vi "Vision Processing.vi"(4 "error in (no error)":errorcluster, 7 "Image Size":T6=enum."320x240") -> ()   [LabVIEW 2015]
doc: "This VI runs in parallel to other tasks. It gets images from the camera, processes them for color or shape and use that information to affect robot behavior."
uses:
  <vilib>/Rock Robotics/WPI/Camera/WPI_CameraImageSize.ctl
  examples/Vision Support Code/Camera Types.ctl
  <vilib>/Rock Robotics/WPI/Camera/WPI_CameraWhite Balance Values.ctl
  <vilib>/Rock Robotics/WPI/Camera/WPI_CameraExposure Values.ctl
  <vilib>/Rock Robotics/WPI/Camera/WPI_CameraFrameRate.ctl
  Robot Global Data.vi
  <vilib>/vision/NI_Vision_Development_Module.lvlib
  <vilib>/Rock Robotics/Network Tables/NT Read Numeric Array.vi
panel:
  in  "Right Boundary":dbl=0.07
  in  "Left Boundary":dbl=-0.07
  out "Centering Command":enum16{"NULL", "RIGHT", "LEFT", "CENTER"}(ring)
  out "Horizontal Centering":dbl
  out "fps":dbl
  in  "LED Color":T1={"Hue"={97.8946764540238, 78.89044183841362}, "Sat"={182.14285714285714, 255.0}, "Val"={106.25, 255.0}} {"Hue" scale=0.0..255.0 scale format="%#_3g"}
  out "Qualified Particles":i32
  in  "Score Threshold":dbl=75.0
  in  "Aspect Fudge Factor":dbl=1.0
  in  "Min Score Threshold":i32=75
  in  "Camera Type":T2=enum."1011"
  in  "Emphasize Limit Tests":bool=TRUE
  out "Masked":T3(plugin-control)
  in  "Display Mask":bool=TRUE
  out "Original Image":T3(plugin-control)
  in  "Display Original":bool=TRUE
  out "Sorted Particle Scores":T4(array[cluster]) {"Moment Factor" format="%#_3g"; "Aspect Ratio" format="%#_3g"; "Area to CH" format="%#_3g"; "X" format="%#_3g"; "Y" format="%#_3g"}
  out "Highest Avg Score":dbl
  out "Detected Targets":T5(array[cluster]) {"Normalized Rect"."Numeric 5" format="%#_2g"; "Normalized Rect"."Numeric 3" format="%#_2g"; "Normalized Rect"."Numeric 2" format="%#_2g"; "Normalized Rect"."Numeric" format="%#_2g"}
  out "ms to process":u32
  # "Density Profile"
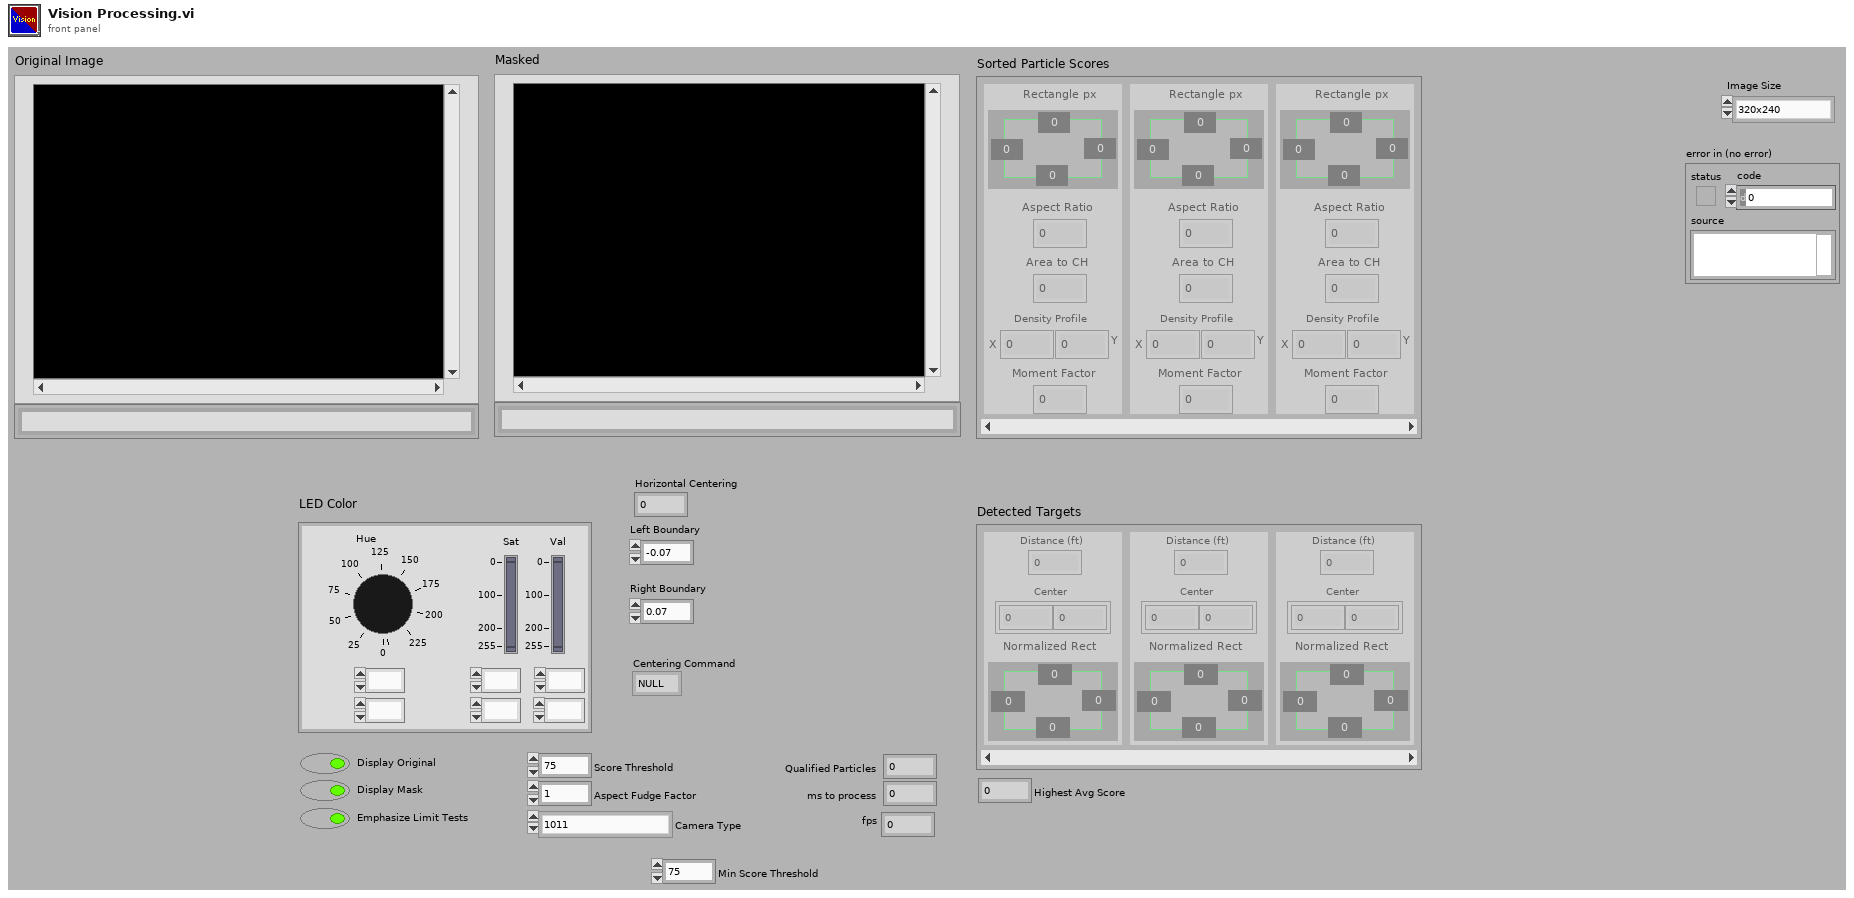
[diagram p1: front panel]
types:
  T1 = cluster{"Hue":cluster{dbl, dbl}, "Sat":cluster{dbl, dbl}, "Val":cluster{dbl, dbl}}
  T2 = typedef "Camera Types.ctl" = enum16{"206", "1011", "1013", "MS HD3000 square", "MS HD3000 640x480"}
  T3 = typedef "IMAQ Image.ctl" = refnum<image>
  T4 = cluster{"Rectangle px":cluster{"Numeric":dbl, "Numeric 2":dbl, "Numeric 3":dbl, "Numeric 5":dbl}, "Aspect Ratio":dbl, "Area to CH":dbl, "X":dbl, "Y":dbl, "Moment Factor":dbl}[]
  T5 = cluster{"Distance (ft)":dbl, "Center":cluster{dbl, dbl}, "Normalized Rect":cluster{"Numeric":dbl, "Numeric 2":dbl, "Numeric 3":dbl, "Numeric 5":dbl}}[]
  T6 = typedef "WPI_CameraImageSize.ctl" = enum16{"640x480", "320x240", "160x120", "Custom"}
  T7 = typedef "Particle Parameters" = i32
  T8 = typedef "WPI_CameraFrameRate.ctl" = u32
  T9 = typedef "WPI_CameraExposure Values.ctl" = enum16{"Auto", "Flicker-free 50 Hz", "Flicker-free 60 Hz", "Hold current", "Custom"}
  T10 = typedef "WPI_CameraWhite Balance Values.ctl" = enum16{"Auto", "Fixed indoor", "Fixed outdoor 1", "Fixed outdoor 2", "Fixed fluorescent 1", "Fixed fluorescent 2", "Hold current", "Custom"}
  T11 = typedef "Image Type" = u32
  T12 = typedef "WPI_CameraDevRef.ctl" = cluster{"Camera Address":string, "CameraStatus":errorcluster}
  T13 = cluster{"Numeric Array[0]":dbl, "Numeric Array[1]":dbl, "Numeric Array[2]":dbl, "Numeric Array[3]":dbl, "Numeric Array[4]":dbl, "Numeric Array[5]":dbl, "Numeric Array[6]":dbl, "Numeric Array[7]":dbl, "Numeric Array[8]":dbl}
  T14 = cluster{"Bounding box":cluster{"left":dbl, "top":dbl, "right":dbl, "bottom":dbl}, "Aspect Ratio":dbl, "Area to CH":dbl, "X Mask":dbl, "Y Mask":dbl, "Moment":dbl}[]
  T15 = cluster{"Rectangle":cluster{"Numeric":dbl, "Numeric 2":dbl, "Numeric 3":dbl, "Numeric 5":dbl}, "L":dbl, "Area to CH":dbl, "X":dbl, "Y":dbl, "Moment Factor":dbl}[]
  T16 = cluster{"Found Targets[0]":cluster{"Distance (ft)":dbl, "Center":cluster{dbl, dbl}, "Normalized Rect":cluster{"Numeric":dbl, "Numeric 2":dbl, "Numeric 3":dbl, "Numeric 5":dbl}}, "Found Targets[1]":cluster{"Distance (ft)":dbl, "Center":cluster{dbl, dbl}, "Normalized Rect":cluster{"Numeric":dbl, "Numeric 2":dbl, "Numeric 3":dbl, "Numeric 5":dbl}}, "Found Targets[2]":cluster{"Distance (ft)":dbl, "Center":cluster{dbl, dbl}, "Normalized Rect":cluster{"Numeric":dbl, "Numeric 2":dbl, "Numeric 3":dbl, "Numeric 5":dbl}}, "Found Targets[3]":cluster{"Distance (ft)":dbl, "Center":cluster{dbl, dbl}, "Normalized Rect":cluster{"Numeric":dbl, "Numeric 2":dbl, "Numeric 3":dbl, "Numeric 5":dbl}}, "Found Targets[4]":cluster{"Distance (ft)":dbl, "Center":cluster{dbl, dbl}, "Normalized Rect":cluster{"Numeric":dbl, "Numeric 2":dbl, "Numeric 3":dbl, "Numeric 5":dbl}}, "Found Targets[5]":cluster{"Distance (ft)":dbl, "Center":cluster{dbl, dbl}, "Normalized Rect":cluster{"Numeric":dbl, "Numeric 2":dbl, "Numeric 3":dbl, "Numeric 5":dbl}}, "Found Targets[6]":cluster{"Distance (ft)":dbl, "Center":cluster{dbl, dbl}, "Normalized Rect":cluster{"Numeric":dbl, "Numeric 2":dbl, "Numeric 3":dbl, "Numeric 5":dbl}}, "Found Targets[7]":cluster{"Distance (ft)":dbl, "Center":cluster{dbl, dbl}, "Normalized Rect":cluster{"Numeric":dbl, "Numeric 2":dbl, "Numeric 3":dbl, "Numeric 5":dbl}}, "Found Targets[8]":cluster{"Distance (ft)":dbl, "Center":cluster{dbl, dbl}, "Normalized Rect":cluster{"Numeric":dbl, "Numeric 2":dbl, "Numeric 3":dbl, "Numeric 5":dbl}}}
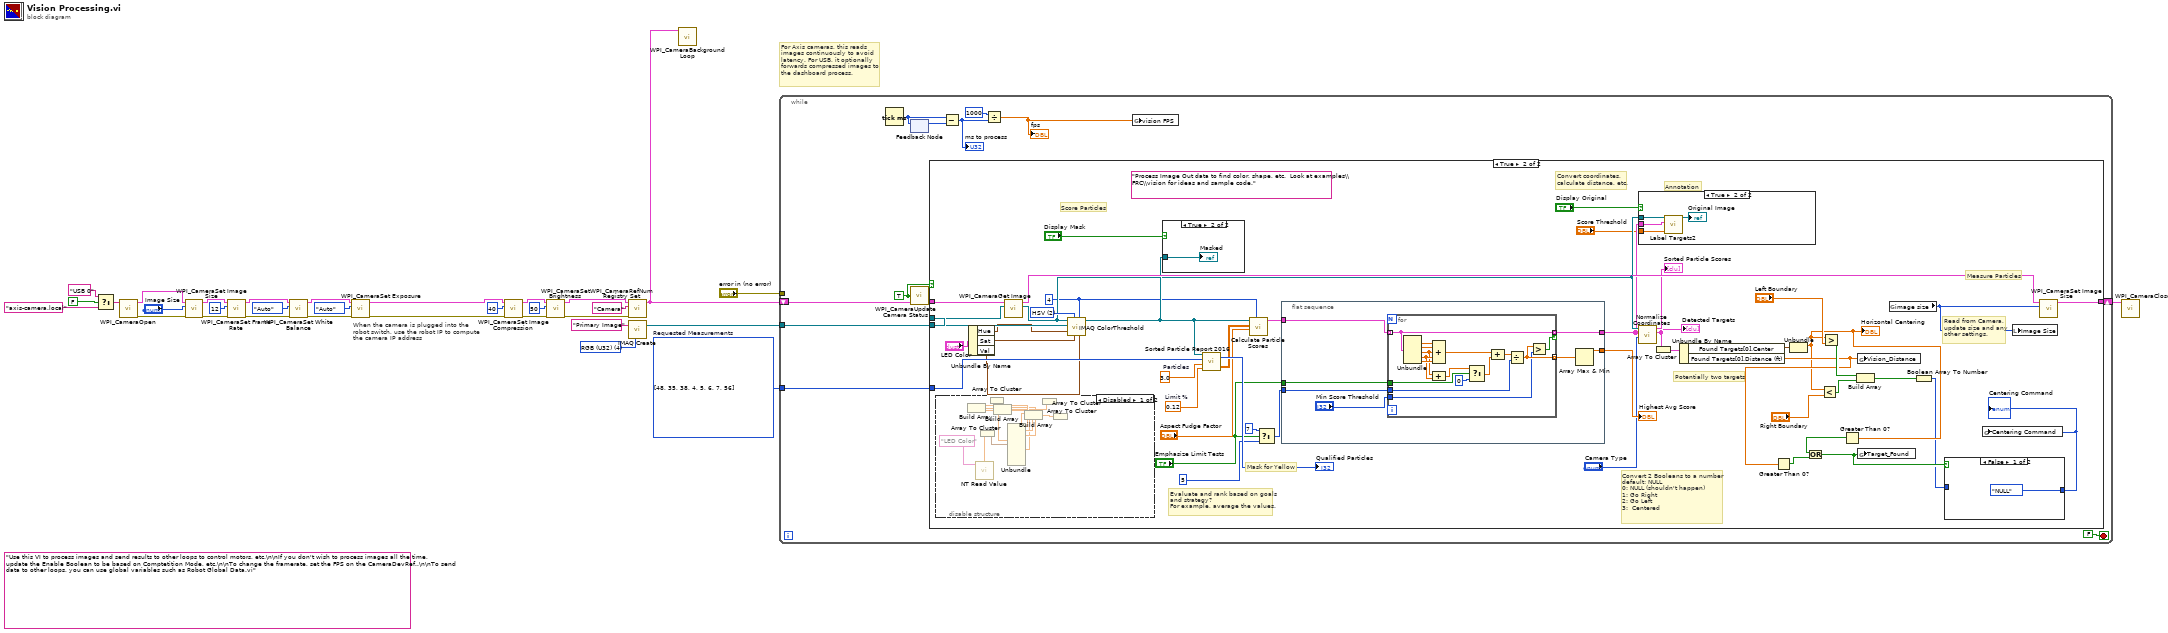
[diagram p0: block diagram]
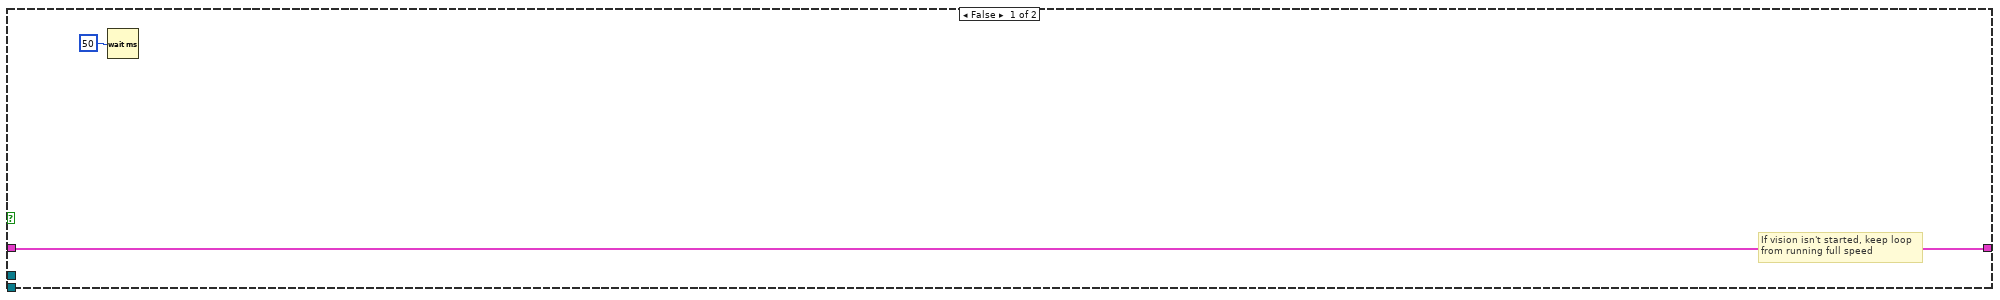
[diagram p2: hidden frame]
diagram:
  w1 = T7[] [48, 35, 38, 4, 5, 6, 7, 56] items=["Center of Mass X", "Center of Mass Y", "First Pixel X", "First Pixel Y", "Bounding Rect Left", "Bounding Rect Top", "Bounding Rect Right", "Bounding Rect Bottom", "Max Feret Diameter Start X", "Max Feret Diameter Start Y", "Max Feret Diameter End X", "Max Feret Diameter End Y", "Max Horiz. Segment Length Left", "Max Horiz. Segment Length Right", "Max Horiz. Segment Length Row", "-", "Bounding Rect Width", "Bounding Rect Height", "Bounding Rect Diagonal", "Perimeter", "Convex Hull Perimeter", "Holes' Perimeter", "Max Feret Diameter", "Equivalent Ellipse Major Axis", "Equivalent Ellipse Minor Axis", "Equivalent Ellipse Minor Axis (Feret)", "Equivalent Rect Long Side", "Equivalent Rect Short Side", "Equivalent Rect Diagonal", "Equivalent Rect Short Side (Feret)", "Average Horiz. Segment Length", "Average Vert. Segment Length", "Hydraulic Radius", "Waddel Disk Diameter", "-", "Area", "Holes' Area", "Particle & Holes' Area", "Convex Hull Area", "Image Area", "-", "Number of Holes", "Number of Horiz. Segments", "Number of Vert. Segments", "-", "Orientation", "Max Feret Diameter Orientation", "-", "% Area/Image Area", "% Area/(Particle & Holes' Area)", "Ratio of Equivalent Ellipse Axes", "Ratio of Equivalent Rect Sides", "-", "Elongation Factor", "Compactness Factor", "Heywood Circularity Factor", "Type Factor", "-", "Sum X", "Sum Y", "Sum XX", "Sum XY", "Sum YY", "Sum XXX", "Sum XXY", "Sum XYY", "Sum YYY", "-", "Moment of Inertia XX", "Moment of Inertia XY", "Moment of Inertia YY", "Moment of Inertia XXX", "Moment of Inertia XXY", "Moment of Inertia XYY", "Moment of Inertia YYY", "Norm. Moment of Inertia XX", "Norm. Moment of Inertia XY", "Norm. Moment of Inertia YY", "Norm. Moment of Inertia XXX", "Norm. Moment of Inertia XXY", "Norm. Moment of Inertia XYY", "Norm. Moment of Inertia YYY", "Hu Moment 1", "Hu Moment 2", "Hu Moment 3", "Hu Moment 4", "Hu Moment 5", "Hu Moment 6", "Hu Moment 7"]  # Requested Measurements
  (unwired) "Use this VI to process images and send results to other loops to control motors, etc.\n\nIf you don't wish to process images all the time, update the Enable Boolean to be based on Comptetition Mode, etc.\n\nTo change the framerate, set the FPS on the CameraDevRef..\n\nTo send data to other loops, you can use global variables such as Robot Global Data.vi"
  w32 = T11 4 items=["Grayscale (U8)", "Grayscale (I16)", "Grayscale (SGL)", "Complex (CSG)", "RGB (U32)", "HSL (U32)", "RGB (U64)"] ("Image Type")
  # "When the camera is plugged into the\nrobot switch, use the robot IP to compute\nthe camera IP address"
  # "For Axis cameras, this reads\nimages continuously to avoid\nlatency. For USB, it optionally\nforwards compressed images to\nthe dashboard process."
  n1 = Select(t="USB 0" ("format string"), s=FALSE ("dot notation? (F)"), f="axis-camera.local" ("format string")) -> (s? t:f=w3:string)
  n2 = call <vilib>:"WPI_CameraOpen.vi"("Camera Address"=w3) -> ("error out"=w20:errorcluster, "CameraDevRef"=w21:T12)  [unwired: 1 in, 8 out]
  n3 = call <vilib>:"WPI_CameraSet Image Size.vi"("error in (no error)"=w20, "Image Size"="Image Size", "CameraDevRef"=w21) -> ("error out"=w19:errorcluster, "CameraDevRef Out"=w22:T12)  [unwired: 1 in, 6 out]
  n4 = call <vilib>:"WPI_CameraSet Frame Rate.vi"("error in (no error)"=w19, "Frame Rate (fps)"=T8 12, "CameraDevRef"=w22) -> ("error out"=w18:errorcluster, "CameraDevRef Out"=w24:T12)  [unwired: 7 out]
  n5 = call <vilib>:"WPI_CameraSet White Balance.vi"("error in (no error)"=w18, "White Balance"=WPI_CameraWhite_Balance_Values."Auto", "CameraDevRef"=w24) -> ("error out"=w17:errorcluster, "CameraDevRef Out"=w23:T12)  [unwired: 1 in, 6 out]
  n6 = call <vilib>:"WPI_CameraSet Exposure.vi"("error in (no error)"=w17, "Exposure"=WPI_CameraExposure_Values."Auto", "CameraDevRef"=w23) -> ("error out"=w16:errorcluster, "CameraDevRef Out"=w26:T12)  [unwired: 1 in, 6 out]
  n7 = call <vilib>:"WPI_CameraSet Image Compression.vi"("error in (no error)"=w16, "Compression"=40, "CameraDevRef"=w26) -> ("error out"=w15:errorcluster, "CameraDevRef Out"=w25:T12)  [unwired: 7 out]
  n8 = call <vilib>:"WPI_CameraSet Brightness.vi"("error in (no error)"=w15, "Brightness"=50, "CameraDevRef"=w25) -> ("error out"=w13:errorcluster, "CameraDevRef Out"=w14:T12)  [unwired: 7 out]
  n9 = call <vilib>:"WPI_CameraRefNum Registry Set.vi"("error in (no error)"=w13, "refnum name"="Camera", "CameraDevRef"=w14) -> ("CameraDevRef"=w9:T12)  [unwired: 1 in, 7 out]
  n10 = call "IMAQ Create"("Image Name"="Primary Image", "Image Type"=w32) -> ("New Image"=w30:T3)  [unwired: 2 in, 2 out]
  n11 = call <vilib>:"WPI_CameraBackground Loop.vi"("CameraDevRef"=w9) -> ()  [unwired: 11 in]
  n12 = while {
    shift-right: [w35] -> w7
    shift-left: w9 -> [w38]
    tunnel: w30 -> [w37]
    tunnel: "error in (no error)" -> [_]
    tunnel: w1 -> [w36]
    stop <- FALSE stop-if-true
    w34 = TRUE
    n13 = Tick Count (ms)() -> (millisecond timer value=w42:u32)
    n14 = feedback #1() -> (w43:u32)  [unwired: 1 in]
    n15 = feedback-in #1(w42) -> ()
    n16 = call <vilib>:"WPI_CameraUpdate Camera Status.vi"("CameraDevRef In"=w38, "Enable Vision"=w34) -> ("CameraDevRef Out"=w41:T12)  [unwired: 3 in]
    n17 = case shown="True" w34 {
      tunnel: w37 -> [_ w93]
      tunnel: w36 -> [_ w92]
      tunnel: w41 -> [w45 w88]
      tunnel: w37 -> [_ w87]
      tunnel: [w45 w85] -> w35
      frame False {
        # "If vision isn't started, keep loop\nfrom running full speed"
        n18 = Wait (ms)(milliseconds to wait=u32 50) -> ()  [unwired: 1 out]
      }
      frame True {
        w70 = 4 ("Replace Value")
        w82 = u16 2 items=["RGB", "HSL", "HSV", "HSI"] ("Color Mode")
        (unwired) "Process Image Out data to find color, shape, etc.  Look at examples\\FRC\\vision for ideas and sample code."
        w89 = 0.12  # Limit %
        w91 = 3.0  # Particles
        # "Evaluate and rank based on goals\nand strategy?\nFor example, average the values."
        # "Potentially two targets"
        # "Convert 2 Booleans to a number\ndefault: NULL\n0: NULL (shouldn't happen)\n1: Go Right\n2: Go Left\n3:  Centered"
        # "Read from Camera,\nupdate size and any\nother settings."
        # "Measure Particles"
        # "Convert coordinates,\ncalculate distance, etc."
        # "Annotation"
        # "Score Particles"
        # "Mask for Yellow"
        n19 = disable-structure shown="Disabled" {
          frame Disabled {
            n20 = call-poly <vilib>:"NT Read Value.vi"("Name"="LED Color") -> ("Numeric Array"=w105:dbl[])  [unwired: 9 in, 1 out]
            n21 = Array To Cluster(array=w105) -> (cluster=w104:T13)
            n22 = Unbundle(w104) -> ("Numeric Array[0]"=w103:dbl, "Numeric Array[1]"=w102:dbl, "Numeric Array[2]"=w99:dbl, "Numeric Array[3]"=w98:dbl, "Numeric Array[4]"=w96:dbl, "Numeric Array[5]"=w95:dbl)  [unwired: 3 out]
            n23 = Build Array(w103, w102) -> (w101:dbl[])
            n24 = Array To Cluster(array=w101) -> ()  [unwired: 1 out]
            n25 = Build Array(w99, w98) -> (w100:dbl[])
            n26 = Build Array(w96, w95) -> (w97:dbl[])
            n27 = Array To Cluster(array=w100) -> ()  [unwired: 1 out]
            n28 = Array To Cluster(array=w97) -> ()  [unwired: 1 out]
          }
          frame Enabled {
          }
        }
        n29 = Unbundle By Name("LED Color") -> ("Hue"=w49:cluster{dbl, dbl}, "Sat"=w50:cluster{dbl, dbl}, "Val"=w48:cluster{dbl, dbl})
        n30 = call <vilib>:"WPI_CameraGet Image.vi"("Image"=w87, "CameraDevRef"=w88) -> ("Image Out"=w73:T3, "CameraDevRef Out"=w86:T12)  [unwired: 7 in, 1 out]
        n31 = call "IMAQ ColorThreshold"("Blue or Luma or Val or Inten Range"=w48, "Replace Value"=w70, "Green or Sat Range"=w50, "Color Mode"=w82, "Red or Hue Range"=w49, "Image Dst"=w93, "Image Src"=w73) -> ("Image Dst Out"=w81:T3)  [unwired: 3 in, 1 out]
        n32 = case shown="True" "Display Mask" {
          tunnel: w81 -> [_ w112]
          frame False {
          }
          frame True {
            "Masked" <- w112
          }
        }
        n33 = call "Sorted Particle Report 2016.vi"("Min Area Size %"=w89, "Particle Count Limit"=w91, "Pixel Measurements"=w92, "Image in"=w81) -> ("Sorted Data"=w80:dbl[][], "Particles"=→"Qualified Particles":i32)
        n34 = call "Calculate Particle Scores.vi"("Pixel Value"=w70, "Aspect Fudge Factor"="Aspect Fudge Factor", "Sorted Data"=w80, "Image in"=w81) -> ("Scores"=w78:T14)  [unwired: 7 in]
        n35 = Select(t=7, s="Emphasize Limit Tests", f=5) -> (s? t:f=w76:i32)
        n36 = flat-sequence {
          tunnel: w78 -> [w118]
          tunnel: w76 -> [w116]
          tunnel: [w119] -> w75
          tunnel: [w113] -> w72
          tunnel: "Emphasize Limit Tests" -> [w117]
          frame #0 {
            n37 = for {
              tunnel: w118 -> [w133] mode=indexing
              tunnel: [w133] -> w113 mode=indexing if=w132
              tunnel: [w131] -> w114 mode=indexing
              tunnel: w116 -> [w130]
              tunnel: "Min Score Threshold" -> [w129]
              tunnel: w117 -> [w122]
              n38 = Unbundle(w133) -> ("Aspect Ratio"=w135:dbl, "Area to CH"=w134:dbl, "X Mask"=w124:dbl, "Y Mask"=w125:dbl, "Moment"=w126:dbl)  [unwired: 1 out]
              n39 = Compound Arithmetic op=ADD(w135, w134, w124, w125, w126) -> (w128:dbl)
              n40 = Compound Arithmetic op=ADD(w124, w125) -> (w123:dbl)
              n41 = Select(t=w123, s=w122, f=0) -> (s? t:f=w121:dbl)
              n42 = Compound Arithmetic op=ADD(w128, w121) -> (w127:dbl)
              n43 = Divide(x=w127, y=w130) -> (x/y=w131:dbl)
              n44 = Greater?(x=w131, y=w129) -> (0:w132:bool)
            }
            n45 = Array Max & Min(array=w114) -> (max value=w119:dbl)  [unwired: 3 out]
          }
        }
        n46 = case shown="True" "Display Original" {
          tunnel: w73 -> [_ w111]
          tunnel: w72 -> [_ w109]
          tunnel: "Score Threshold" -> [_ w108]
          frame False {
          }
          frame True {
            n47 = call "Label Targets2.vi"("Score Threshold"=w108, "Targets"=w109, "Image in"=w111) -> ("Image out"=→"Original Image":T3)  [unwired: 8 in]
          }
        }
        n48 = call "Normalize Coordinates.vi"("Camera Type"="Camera Type", "Targets"=w72, "Image in"=w73) -> ("Found Targets"=w59:T5, "Sorted Scores"=→"Sorted Particle Scores":T15)  [unwired: 7 in]
        "Detected Targets" <- w59
        n49 = Array To Cluster(array=w59) -> (cluster=w65:T16)
        n50 = Unbundle By Name(w65) -> ("Found Targets[0].Center"=w66:cluster{dbl, dbl}, "Found Targets[0].Distance (ft)"=w58:dbl)
        n51 = Greater Than 0?(x=w58) -> (x > 0?=w56:bool)
        n52 = Unbundle(w66) -> (w57:dbl)  [unwired: 1 out]
        "Horizontal Centering" <- w57
        n53 = Less?(x=w57, y="Right Boundary") -> (x < y?=w63:bool)
        n54 = Greater?(x=w57, y="Left Boundary") -> (0:w62:bool)
        n55 = Greater Than 0?(x=w57) -> (x > 0?=w55:bool)
        n56 = Or(x=w55, y=w56) -> (x .or. y?=w54:bool)
        n57 = Build Array(w62, w63) -> (w61:bool[])
        n58 = global write "Robot Global Data.vi" "Vision_Distance"(w58) -> ()
        n59 = global write "Robot Global Data.vi" "Target_Found"(w54) -> ()
        n60 = global read "Robot Global Data.vi" "image size"() -> (w69:T6)
        n61 = Boolean Array To Number(Boolean array=w61) -> (number=w53:u32)
        n62 = case shown="False" w54 {
          tunnel: w53 -> [_ w107]
          tunnel: [enum16{"NULL"}."NULL" w107] -> w52
          frame False {
          }
          frame True {
          }
        }
        "Centering Command" <- w52
        n63 = global write "Robot Global Data.vi" "Centering Command"(w52) -> ()
        n64 = local write "Image Size"(w69) -> ()
        n65 = call <vilib>:"WPI_CameraSet Image Size.vi"("Image Size"=w69, "CameraDevRef"=w86) -> ("CameraDevRef Out"=w85:T12)  [unwired: 2 in, 7 out]
        "Highest Avg Score" <- w75
      }
    }
    n66 = Subtract(x=w42, y=w43) -> (x-y=w40:u32)
    "ms to process" <- w40
    n67 = Divide(x=1000 ("Brightness"), y=w40) -> (x/y=w33:dbl)
    "fps" <- w33
    n68 = global write "Robot Global Data.vi" "vision FPS"(w33) -> ()
  }
  n69 = call <vilib>:"WPI_CameraClose.vi"("CameraDevRef"=w7) -> ()  [unwired: 1 in, 10 out]
